vi "Actor Core.vi"(8 "error in":errorcluster, 11 "Admin_Actor in":refnum<class "Admin_Actor.lvclass">) -> (0 "error out":errorcluster, 3 "Actor out":refnum<class "Actor.lvclass">)   [LabVIEW 2015, in "Admin_Actor.lvlib" / "Admin_Actor.lvclass"]
doc: "(<B>Filename</B>: Actor Framework.lvlib:Actor.lvclass:Actor Core.vi)\n\nReceives messages to the actor, reacts to them, and initiates any error handling that may shut the actor down.\n\nDescendant classes may override this VI to append parallel tasks for the actor to complete while it handles messages. Overrides use the Call Parent Method node."
uses:
  Admin_Actor.lvclass
  <vilib>/ActorFramework/Actor/Actor.lvclass
  <vilib>/ActorFramework/Actor/Actor.lvclass/Actor.ctl
  <vilib>/ActorFramework/Message Enqueuer/Message Enqueuer.lvclass/Message Enqueuer.ctl
  <vilib>/ActorFramework/Stop Msg/Stop Msg.lvclass/Stop Msg.ctl
  Admin_Actor Messages/SwitchOption Msg/SwitchOption Msg.lvclass
  User_Actor/Member_Actor Messages/SwitchOption Msg/SwitchOption Msg.lvclass/SwitchOption Msg.ctl
  <vilib>/ActorFramework/Message Enqueuer/Init from Existing Queue.vi
  <vilib>/ActorFramework/Message Enqueuer/Enqueue Critical.vi
  <vilib>/ActorFramework/Message Enqueuer/Enqueue.vi
  <vilib>/ActorFramework/Message Priority Queue/Priority Enqueue.vi
  <vilib>/ActorFramework/Message Enqueuer/Message Enqueuer.lvclass
  <vilib>/ActorFramework/Stop Msg/Stop Msg.lvclass
  User_Actor/User_Actor/User_Actor.lvclass
  User_Actor/Member_Actor Messages/SwitchOption Msg/SwitchOption Msg.lvclass
panel:
  in  "提示":string
  in  "Attendance":bool
  in  "ExcuseNotes":bool
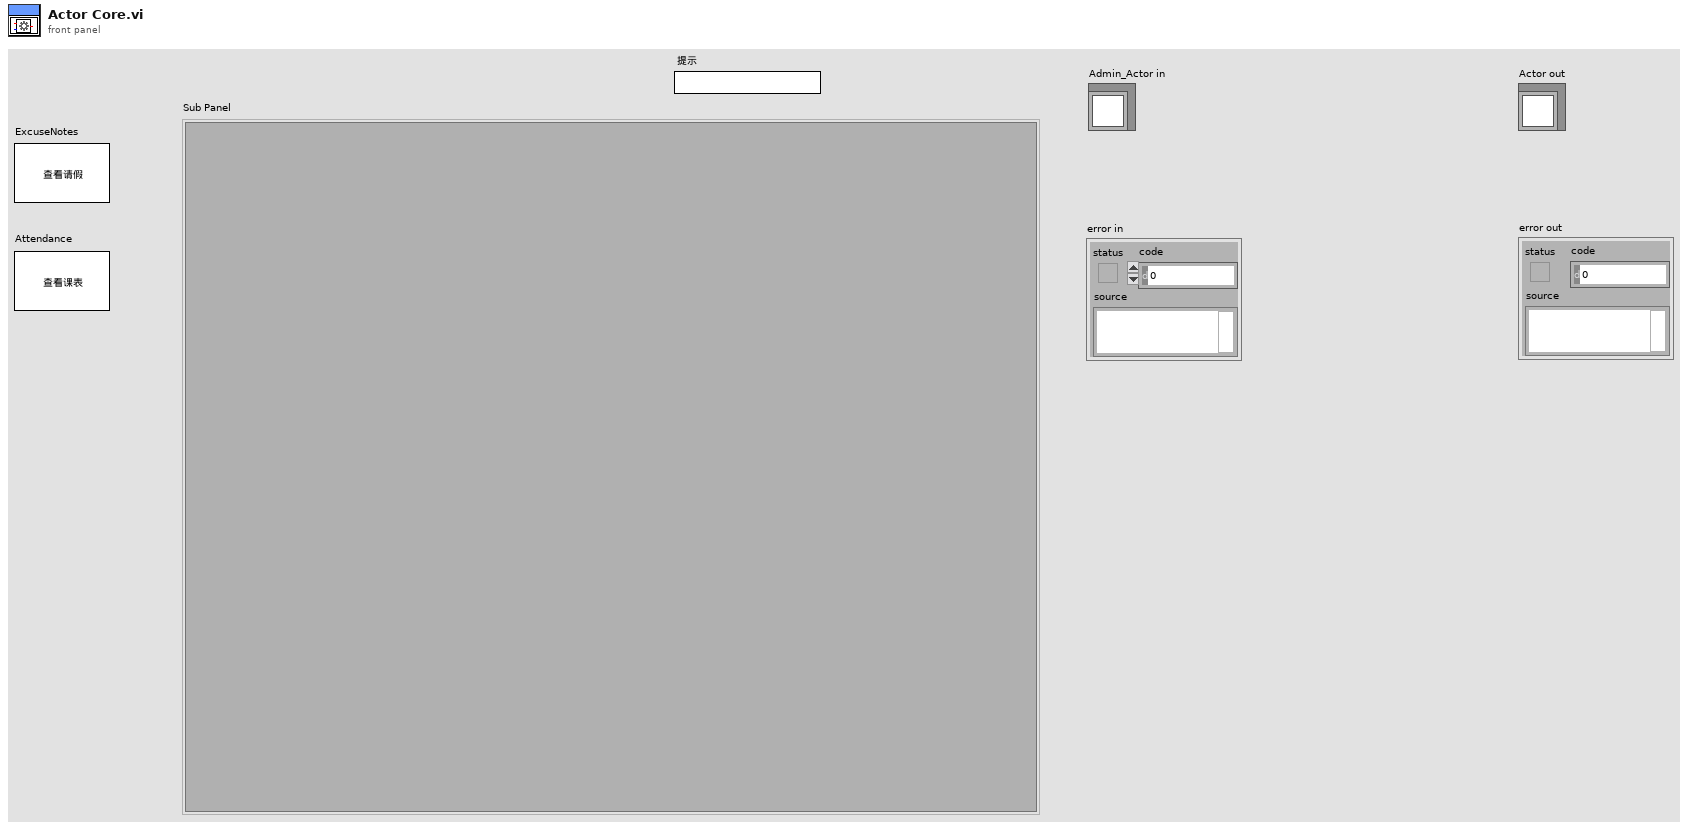
[diagram p1: front panel]
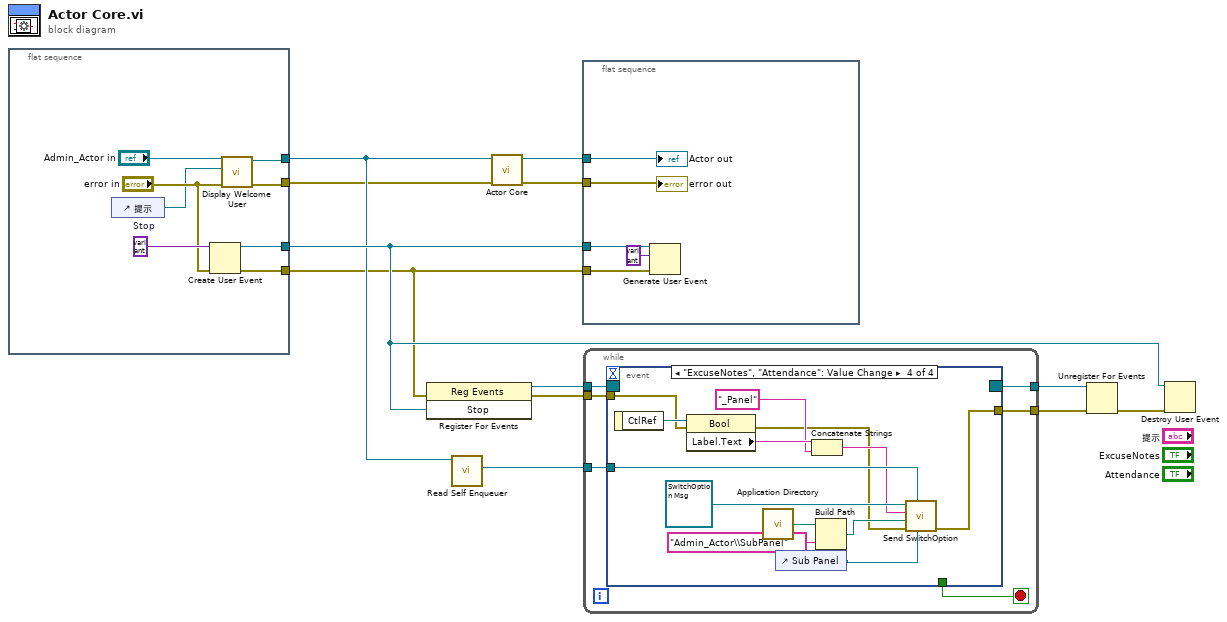
[diagram p0: block diagram]
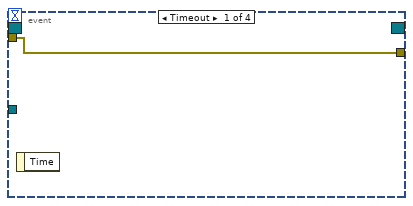
[diagram p2: hidden frame]
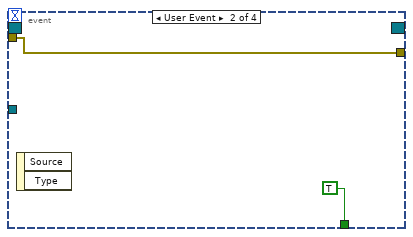
[diagram p3: hidden frame]
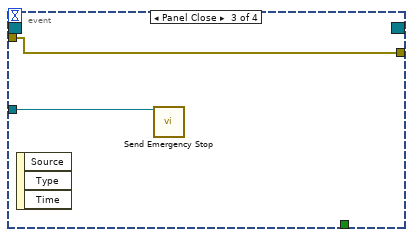
[diagram p4: hidden frame]
diagram:
  n1 = flat-sequence {
    tunnel: [w14] -> w3
    tunnel: [w13] -> w7
    tunnel: [w19] -> w11
    tunnel: [w18] -> w5
    frame #0 {
      w20 = variant  # Stop
      n2 = control-ref of="提示"() -> (w15:refnum<vi>)
      n3 = Create User Event(user event datatype=w20, error in="error in") -> (user event=w19:refnum<user-event>, error out=w18:errorcluster)
      n4 = call "Display Welcome User.vi"("error in (no error)"="error in", "Sign(Ref)"=w15, "Admin_Actor in"="Admin_Actor in") -> ("error out"=w14:errorcluster, "Admin_Actor out"=w13:refnum<class "Admin_Actor.lvclass">)  [unwired: 7 in]
    }
  }
  n5 = register-events(error in=w5, w11) -> (reference out=w4:refnum<event-registration>, error out=w6:errorcluster)  [unwired: 1 in]
  n6 = call <vilib>:"Read Self Enqueuer.vi"("Actor"=w7) -> ("Self Enqueuer"=w8:refnum<class "Message Enqueuer.lvclass">)  [unwired: 10 in]
  n7 = call-parent "Actor Core.vi"("error in"=w3, "Actor in"=w7) -> ("error out"=w1:errorcluster, "Actor out"=w2:refnum<class "Actor.lvclass">)  [unwired: 8 in]
  n8 = flat-sequence {
    tunnel: w1 -> [w22]
    tunnel: w2 -> [w21]
    tunnel: w11 -> [w25]
    tunnel: w5 -> [w24]
    frame #0 {
      n9 = Generate User Event(user event=w25, event data cluster=variant ("event data"), error in=w24) -> ()  [unwired: 1 in, 2 out]
      "error out" <- w22
      "Actor out" <- w21
    }
  }
  n10 = while {
    tunnel: w4 -> [w31]
    tunnel: w6 -> [w30]
    tunnel: w8 -> [w29]
    tunnel: [w27] -> w9
    tunnel: [w26] -> w10
    stop <- w28 stop-if-true
    n11 = event shown="[3] \"ExcuseNotes\", \"Attendance\": Value Change" {
      selector: w31 -> [_ _ _ _]
      dyn-events: [_ _ _ _] -> w27
      timeout: _ -> [_ _ _ _]
      tunnel: w30 -> [w32 w33 w35 w45]
      tunnel: w29 -> [_ _ w36 w48]
      tunnel: [_ TRUE _ _] -> w28
      tunnel: [w32 w33 w35 w38] -> w26
      event Timeout {
        n12 = event-data() -> ()  [unwired: 1 in, 1 out]
      }
      event User Event {
        n13 = event-data() -> ()  [unwired: 1 in, 2 out]
      }
      event Panel Close {
        n14 = event-data() -> ()  [unwired: 1 in, 3 out]
        n15 = call <vilib>:"Send Emergency Stop.vi"("Message Enqueuer"=w36) -> ()  [unwired: 10 in, 1 out]
      }
      event "ExcuseNotes", "Attendance": Value Change {
        n16 = event-data() -> ("CtlRef"=w46:refnum<vi>)  [unwired: 1 in]
        n17 = property class="Bool"(reference=w46, error in=w45) -> (error out=w39:errorcluster, "Label.Text"=w47:string)  [unwired: 1 out]
        n18 = call <vilib>:"Application Directory.vi"() -> ("Application Directory"=w41:path)
        n19 = control-ref of="Sub Panel"() -> (w37:refnum<vi>)
        n20 = Concatenate Strings(w47, "_Panel" ("string")) -> (w43:string)
        n21 = Build Path(base path=w41, name or relative path="Admin_Actor\\SubPanel") -> (appended path=w40:path)
        n22 = call "Send SwitchOption.vi"("SubPanelRef"=w37, "Message Enqueuer"=w48, "error in (no error)"=w39, "Base Path"=w40, "ThreadName(\"\")"=w43, "Message Type"=refnum<class "SwitchOption Msg.lvclass"> refnum ("Admin_Actor.lvlib:SwitchOption Msg.lvclass")) -> ("error out"=w38:errorcluster)  [unwired: 5 in]
      }
    }
  }
  n23 = Unregister For Events(event registration refnum=w9, error in=w10) -> (error out=w12:errorcluster)
  n24 = Destroy User Event(user event=w11, error in=w12) -> ()  [unwired: 1 out]
